vi "append_ring_buffer.vi"(7 "max len":i32=1000, 9 "xyz":T2, 11 "data in":T1) -> (3 "data out":T1)   [LabVIEW 2019, in "Nano33BLE-TiltCompensationSupport.lvlib"]
uses:
  types/xyz_array.ctl
  types/xyz.ctl
  Nano33BLE-TiltCompensationSupport.lvlib
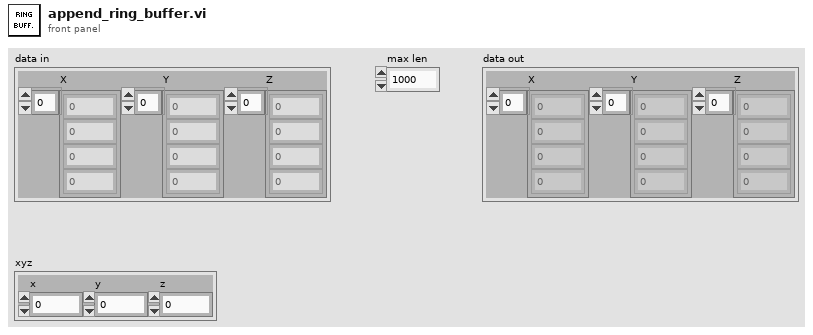
[diagram p1: front panel]
types:
  T1 = typedef "Nano33BLE-TiltCompensationSupport.lvlib/xyz_array.ctl" = cluster{"X":dbl[], "Y":dbl[], "Z":dbl[]}
  T2 = typedef "Nano33BLE-TiltCompensationSupport.lvlib/xyz.ctl" = cluster{"x":dbl, "y":dbl, "z":dbl}
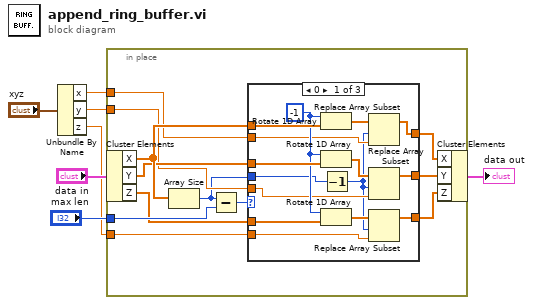
[diagram p0: block diagram]
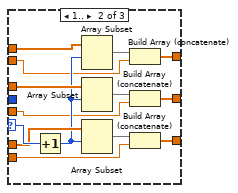
[diagram p2: hidden frame]
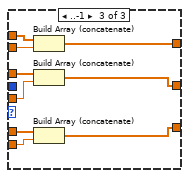
[diagram p3: hidden frame]
diagram:
  n1 = Unbundle By Name("xyz") -> ("x"=w4:dbl, "y"=w3:dbl, "z"=w2:dbl)
  n2 = in-place {
    in-place-border: "max len" -> [w19]
    in-place-border: w4 -> [w14]
    in-place-border: w3 -> [w13]
    in-place-border: w2 -> [w12]
    n3 = in-place-cluster #1("data in") -> ("X"=w17:dbl[], "Y"=w16:dbl[], "Z"=w15:dbl[])
    n4 = Array Size(array=w17) -> (size(s)=w8:i32)
    n5 = Subtract(x=w8, y=w19) -> (x-y=w18:i32)
    n6 = case shown="0" w18 {
      selector: w18 -> [_ w47 _]
      tunnel: w17 -> [w34 w48 w57]
      tunnel: w16 -> [w32 w46 w56]
      tunnel: w15 -> [w33 w45 w55]
      tunnel: w14 -> [w22 w40 w54]
      tunnel: w13 -> [w23 w39 w53]
      tunnel: w12 -> [w24 w38 w52]
      tunnel: [w27 w37 w51] -> w11
      tunnel: [w26 w36 w50] -> w10
      tunnel: [w25 w35 w49] -> w9
      tunnel: w8 -> [w21 _ _]
      frame 0 {
        w31 = -1 ("n")
        n7 = Rotate 1D Array(1:w34, 2:w31) -> (0:w30:dbl[])
        n8 = Rotate 1D Array(1:w32, 2:w31) -> (0:w29:dbl[])
        n9 = Rotate 1D Array(1:w33, 2:w31) -> (0:w28:dbl[])
        n10 = Decrement(x=w21) -> (x-1=w20:i32)
        n11 = Replace Array Subset(array=w30, new element=w22, index=w20) -> (w27:dbl[])
        n12 = Replace Array Subset(array=w29, new element=w23, index=w20) -> (w26:dbl[])
        n13 = Replace Array Subset(array=w28, new element=w24, index=w20) -> (w25:dbl[])
      }
      frame 1.. {
        n14 = Increment(x=w47) -> (x+1=w44:i32)
        n15 = Array Subset(array=w48, index=w44) -> (w43:dbl[])  [unwired: 1 in]
        n16 = Array Subset(array=w46, index=w44) -> (w42:dbl[])  [unwired: 1 in]
        n17 = Array Subset(array=w45, index=w44) -> (w41:dbl[])  [unwired: 1 in]
        n18 = Build Array (concatenate)(w43, w40) -> (w37:dbl[])
        n19 = Build Array (concatenate)(w42, w39) -> (w36:dbl[])
        n20 = Build Array (concatenate)(w41, w38) -> (w35:dbl[])
      }
      frame ..-1 {
        n21 = Build Array (concatenate)(w57, w54) -> (w51:dbl[])
        n22 = Build Array (concatenate)(w56, w53) -> (w50:dbl[])
        n23 = Build Array (concatenate)(w55, w52) -> (w49:dbl[])
      }
    }
    n24 = in-place-cluster #1("X"=w11, "Y"=w10, "Z"=w9) -> (→"data out":T1)
  }
